vi "写入ini文件.vi"(8 "error in (no error)":errorcluster caption="错误输入（无错误）", 9 "值":string[](array[string]), 10 "名称":string[](array[string]), 11 "configuration file path":path caption="配置文件的路径") -> (0 "error out":errorcluster caption="错误输出")   [LabVIEW 2014]
uses:
  <vilib>/Utility/config.llb/Write Key (String).vi
  <vilib>/Utility/config.llb/NI_LVConfig.lvlib
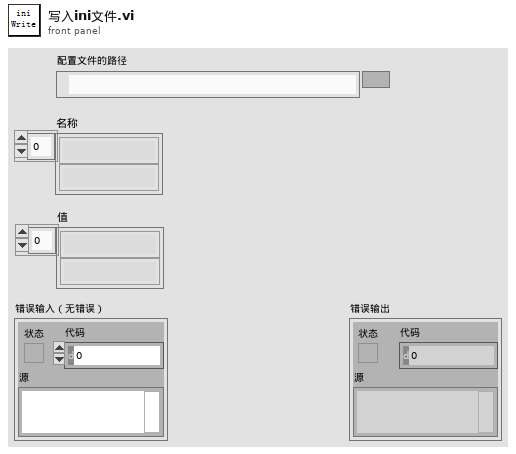
[diagram p1: front panel]
types:
  T1 = typedef "NI_LVConfig.lvlib/Config Data RefNum.ctl" = refnum<k1>
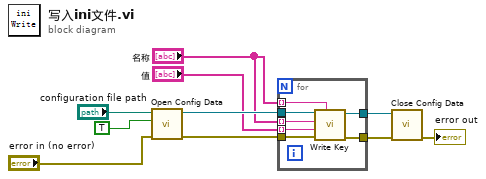
[diagram p0: block diagram]
diagram:
  n1 = call <vilib>:"Open Config Data.vi"("error in (no error)"="error in (no error)", "create file if necessary (T)"=TRUE, "configuration file path"="configuration file path") -> ("error out"=w7:errorcluster, "refnum"=w8:T1)  [unwired: 6 in, 1 out]
  n2 = for {
    tunnel: w8 -> [w17]
    tunnel: w7 -> [w16]
    tunnel: "名称" -> [w15] mode=indexing
    tunnel: "名称" -> [w14] mode=indexing
    tunnel: "值" -> [w13] mode=indexing
    tunnel: [w12] -> w5
    tunnel: [w11] -> w4
    n3 = call-poly <vilib>:"Write Key.vi"("section"=w15, "error in (no error)"=w16, "value"=w13, "key"=w14, "refnum"=w17) -> ("error out"=w11:errorcluster, "refnum out"=w12:T1)  [unwired: 4 in, 1 out]
  }
  n4 = call <vilib>:"Close Config Data.vi"("error in (no error)"=w4, "refnum"=w5) -> ("error out"=→"error out":errorcluster)  [unwired: 8 in, 1 out]
